vi "write_range_command.vi"(11 "Scan Length (Bins)":dbl) -> (3 "Command Out":string)   [LabVIEW 2015]
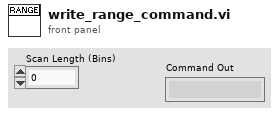
[diagram p1: front panel]
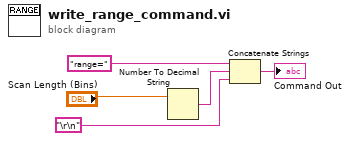
[diagram p0: block diagram]
diagram:
  n1 = Number To Decimal String(number="Scan Length (Bins)") -> (decimal integer string=w3:string)  [unwired: 1 in]
  n2 = Concatenate Strings("range=" ("string"), w3, "\r\n") -> (→"Command Out":string)
